vi "Add Employee to Employee Table.vi"(8 "错误输入（无错误）":errorcluster, 10 "Employee Info":T1, 11 "DataTable":refnum<k24>) -> (0 "错误输出":errorcluster, 3 "DataTable Out":refnum<k24>)   [LabVIEW 2012, in "Employee Info.lvlib"]
uses:
  Employee Info.lvlib
  Employee Info.ctl
  System.Data
  LowLevel/DataGridView.lvlib
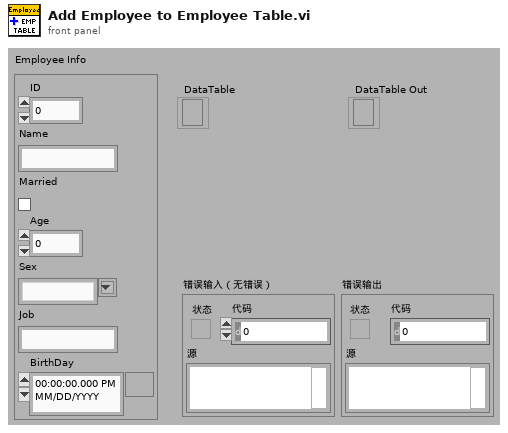
[diagram p1: front panel]
types:
  T1 = typedef "Employee Info.lvlib/Employee Info.ctl" = cluster{"ID":u16, "Name":string, "Married":bool, "Age":u8, "Sex":string, "Job":string, "BirthDay":timestamp}
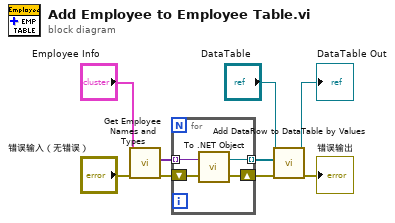
[diagram p0: block diagram]
diagram:
  n1 = call "Get Employee Names and Types.vi"("错误输入（无错误）"="错误输入（无错误）", "Employee Info"="Employee Info") -> ("错误输出"=w5:errorcluster, "Colomn Types"=w6:variant[])  [unwired: 7 in, 1 out]
  n2 = for {
    tunnel: w6 -> [w11] mode=indexing
    shift-right: [w13] -> w3
    shift-left: w5 -> [w12]
    tunnel: [w10] -> w4 mode=indexing
    n3 = call <vilib>:"To .NET Object.vi"("error in (no error)"=w12, "anything"=w11) -> ("error out"=w13:errorcluster, ".NET object"=w10:refnum<k24>)
  }
  n4 = call "Add DataRow to DataTable by Values.vi"("错误输入（无错误）"=w3, "values"=w4, "DataTable"="DataTable") -> ("错误输出"=→"错误输出":errorcluster, "DataTable"=→"DataTable Out":refnum<k24>)  [unwired: 7 in]
